vi "remoteControlArmAndGripper.vi"() -> ()   [LabVIEW 2019]
uses:
  <vilib>/ReMiSYS/ReMiSYS_myRIO-mini/SubVI/gamepadF710/F710.ctl
  <vilib>/ReMiSYS/ReMiSYS_myRIO-mini/SubVI/gamepadF710/stick.ctl
  <vilib>/ReMiSYS/ReMiSYS_myRIO-mini/SubVI/gamepadF710/gamepadF710.lvclass
  <vilib>/Platform/TimedLoop/XDataNode/timing_clust.ctl
  <vilib>/Platform/TimedLoop/XDataNode/nitl_modes.ctl
  <vilib>/Platform/TimedLoop/XDataNode/wakeup.ctl
  <vilib>/ReMiSYS/ReMiSYS_myRIO-mini/SubVI/SYS/servoPort.ctl
  <vilib>/myRIO/Common/Instrument Driver Framework/myRIO v1.0/UART/vis/myRIO v1.0 Close UART.vi
  <vilib>/myRIO/Common/Instrument Driver Framework/Utilities/vis/FPGA Ref Manager.vi
  <vilib>/myRIO/Common/Instrument Driver Framework/myRIO v1.0/myRIO v1.0 Reset FPGA.vi
  <vilib>/myRIO/Common/Instrument Driver Framework/myRIO v1.0/IRQ/vis/myRIO v1.0 IRQ Info FGV.vi
  <vilib>/myRIO/Common/Instrument Driver Framework/myRIO v1.0/IRQ/vis/myRIO v1.0 Timer IRQ Info FGV.vi
  <vilib>/myRIO/Common/Instrument Driver Framework/myRIO v1.0/IRQ/vis/myRIO v1.0 ISR Agent.vi
  <vilib>/myRIO/Instrument Drivers/Utilities/vis/Reset Index.vi
  <vilib>/myRIO/Common/Instrument Driver Framework/myRIO v1.0/Resource Manager/vis/myRIO v1.0 Block Write Resource Manager.vi
  <vilib>/Platform/TimedLoop/XDataNode/XDataNode.xnode
  <vilib>/Platform/TimedLoop/XDataNode/XDNodeRunTimeDep.lvlib
  <vilib>/myRIO/Instrument Drivers/Utilities/Utilities.lvlib
panel:
  out "F710 button info.LogiB":bool
  in  "speed 1~10":dbl=10.0
  out "shooterPitch":dbl
  out "ClipCtrl":bool[](array[boolean])
  out "Speed Array":dbl[](array[numeric])
  in  "stop Control?":bool
  out "F710":T1
  out "ENC [L, R, B] (deg)":dbl[](array[numeric])
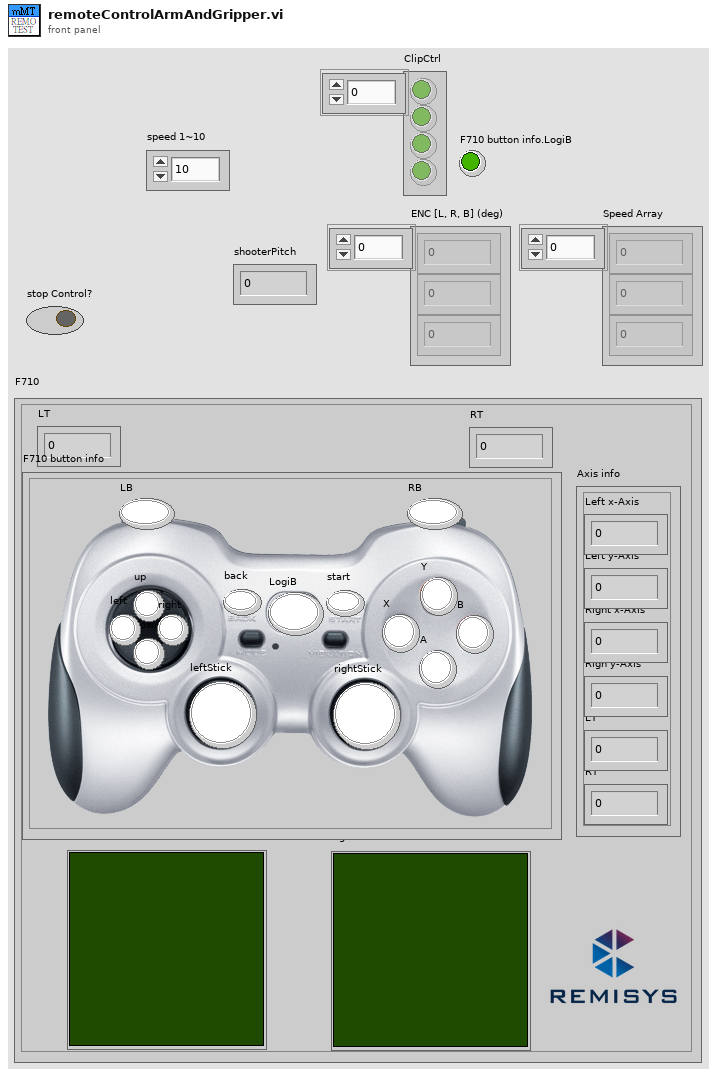
[diagram p1: front panel]
types:
  T1 = typedef "F710.ctl" = cluster{"RT":u8, "LT":u8, "RightStick":T2, "LeftStick":T2, "Axis info":cluster{"Left x-Axis":i8, "Left y-Axis":i8, "Right x-Axis":i8, "Righ y-Axis":i8, "LT":u8, "RT":u8}, "F710 button info":cluster{"RB":bool, "LB":bool, "rightStick":bool, "leftStick":bool, "start":bool, "back":bool, "right":bool, "left":bool, "down":bool, "up":bool, "Y":bool, "X":bool, "B":bool, "A":bool, "LogiB":bool}}
  T2 = typedef "stick.ctl" = cluster{"X":dbl, "Y":dbl}[]
  T3 = typedef "servoPort.ctl" = enum16{"S1", "S2", "S3", "S4", "S5", "S6", "S7", "S8", "S9"}
  T4 = typedef "XDNodeRunTimeDep.lvlib/timing_clust.ctl" = cluster{"Expected End [f-1]":u64, "Actual End [f-1]":u64, "Finished Late? [f-1]":bool, "Expected End [i-1]":u64, "Actual End [i-1]":u64, "Finished Late? [i-1]":bool, "Expected Start [i]":u64, "Actual Start [i]":u64, "Expected Start [f]":u64, "Actual Start [f]":u64, "Source Name":string, "Structure Name":string, "Period":i64, "Deadline":i64, "Offset":i64, "Start":i64, "Priority":i32, "Timeout":i32, "Mode":T5, "Wakeup Reason":T6, "Error":errorcluster, "Source Type":string, "Secondary Source Type":string, "Global End Time":u64, "Global Start Time":u64, "Frame Duration":u64, "Iteration Duration":u64, "Assigned CPU":i32, "I/O Scan Engine Mode":u32}
  T5 = typedef "XDNodeRunTimeDep.lvlib/nitl_modes.ctl" = enum32{"No Change", "Process missed periods, maintain original phase", "Discard missed periods, maintain original phase", "Process missed periods, ignore original phase", "Discard missed periods, ignore original phase"}
  T6 = typedef "XDNodeRunTimeDep.lvlib/wakeup.ctl" = enum32{"Normal", "Aborted", "Asynchronous wakeup", "Timing source error", "Timed loop error", "Timeout"}
  T7 = typedef "miniRef.ctl" = cluster{"Custom FPGA Reference":refnum<k20>, "error out":errorcluster}
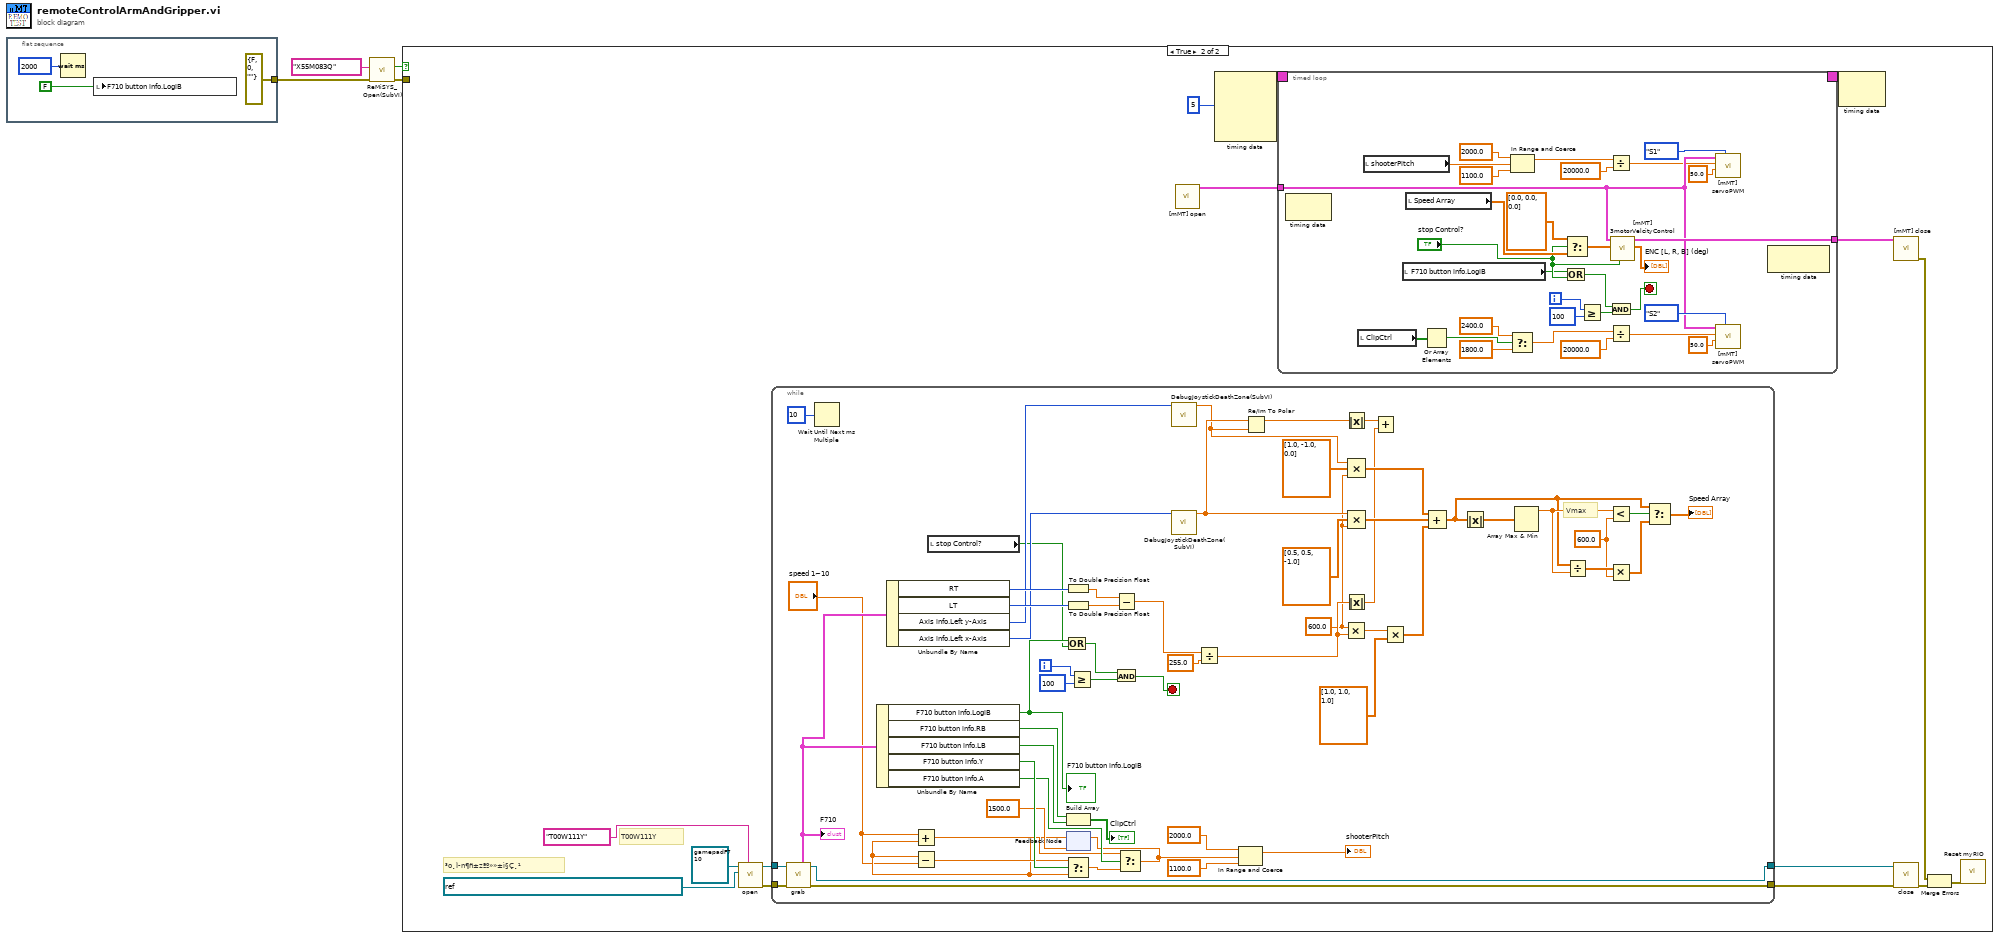
[diagram p0: block diagram]
diagram:
  n1 = flat-sequence {
    tunnel: [errorcluster {"status"=FALSE, "code"=0, "source"=""} ("error in (no error)")] -> w1
    frame #0 {
      n2 = Wait (ms)(milliseconds to wait=u32 2000) -> ()  [unwired: 1 out]
      n3 = local write "F710 button info.LogiB"(FALSE ("x .or. y?")) -> ()
    }
  }
  n4 = call <vilib>:"ReMiSYS_Open(SubVI).vi"("error in (no error)"=w1, "ReMiSYS Key"="X55M083Q") -> ("error out"=w4:errorcluster, "Correct Key?"=w3:bool)  [unwired: 8 in]
  n5 = case shown="True" w3 {
    tunnel: w4 -> [_ _]
    frame False {
    }
    frame True {
      # "T00W111Y"
      # "³o¸Ì­n¶ñ±zªº»»±ì§Ç¸¹"
      n6 = call <vilib>:"open.vi"("INPUT S/N"="T00W111Y", "VISA resource name"=refnum<visa-resource-name> "USB0::0x046D::0xC21F::A6269818::RAW", "gamepadF710 in"=refnum<class "gamepadF710.lvclass"> refnum) -> ("error out"=w13:errorcluster, "gamepadF710 out"=w17:refnum<class "gamepadF710.lvclass">)  [unwired: 7 in]
      n7 = while {
        tunnel: w17 -> [w80]
        tunnel: [w79] -> w16
        tunnel: w13 -> [w52]
        tunnel: [w51] -> w12
        i -> [w26]
        stop <- w23 stop-if-true
        w46 = 600.0 ("y")
        w42 = 600.0 ("tiltScale")
        # "Vmax"
        n8 = call <vilib>:"grab.vi"("error in (no error)"=w52, "gamepadF710 in"=w80) -> ("error out"=w51:errorcluster, "gamepadF710 out"=w79:refnum<class "gamepadF710.lvclass">, "F710"=w67:T1)  [unwired: 6 in]
        "F710" <- w67
        n9 = Wait Until Next ms Multiple(millisecond multiple=u32 10) -> ()  [unwired: 1 out]
        n10 = Unbundle By Name(w67) -> ("F710 button info.LogiB"=w29:bool, "F710 button info.RB"=w66:bool, "F710 button info.LB"=w65:bool, "F710 button info.Y"=w41:bool, "F710 button info.A"=w40:bool)
        "F710 button info.LogiB" <- w29
        n11 = Unbundle By Name(w67) -> ("RT"=w71:u8, "LT"=w69:u8, "Axis info.Left y-Axis"=w63:i8, "Axis info.Left x-Axis"=w62:i8)
        n12 = local read "stop Control?"() -> (w28:bool)
        n13 = Or(x=w29, y=w28) -> (x .or. y?=w27:bool)
        n14 = To Double Precision Float(number=w71) -> (double precision float=w70:dbl)
        n15 = To Double Precision Float(number=w69) -> (double precision float=w68:dbl)
        n16 = Build Array(w66, w65) -> (→"ClipCtrl":bool[])
        n17 = feedback #1(1500.0) -> (w35:dbl)
        n18 = Add(x="speed 1~10", y=w35) -> (x+y=w39:dbl)
        n19 = Subtract(x=w35, y="speed 1~10") -> (x-y=w37:dbl)
        n20 = Select(t=w37, s=w41, f=w35) -> (s? t:f=w38:dbl)
        n21 = Greater Or Equal?(x=w26, y=100) -> (x >= y?=w24:bool)
        n22 = Subtract(x=w70, y=w68) -> (x-y=w61:dbl)
        n23 = And(x=w27, y=w24) -> (x .and. y?=w23:bool)
        n24 = Select(t=w39, s=w40, f=w38) -> (s? t:f=w31:dbl)
        n25 = feedback-in #1(w31) -> ()
        n26 = call <vilib>:"DebugJoystickDeathZone(SubVI).vi"("Axis_Info"=w63) -> ("ValueOut 1~-1"=w58:dbl)  [unwired: 10 in]
        n27 = call <vilib>:"DebugJoystickDeathZone(SubVI).vi"("Axis_Info"=w62) -> ("ValueOut 1~-1"=w59:dbl)  [unwired: 10 in]
        n28 = Divide(x=w61, y=255.0) -> (x/y=w57:dbl)
        n29 = In Range and Coerce(upper limit=2000.0, x=w31, lower limit=1100.0) -> (coerced(x)=→"shooterPitch":dbl)  [unwired: 1 out]
        n30 = Re/Im To Polar(2:w58, 3:w59) -> (1:w56:dbl)  [unwired: 1 out]
        n31 = Multiply(x=w42, y=w57) -> (x*y=w43:dbl)
        n32 = Absolute Value(x=w56) -> (abs(x)=w55:dbl)
        n33 = Absolute Value(x=w57) -> (abs(x)=w54:dbl)
        n34 = Compound Arithmetic op=MULTIPLY(w58, dbl[] [1.0, -1.0, 0.0], w42) -> (w74:dbl[])
        n35 = Compound Arithmetic op=MULTIPLY(w59, dbl[] [0.5, 0.5, -1.0], w42) -> (w73:dbl[])
        n36 = Add(x=w55, y=w54) -> ()  [unwired: 1 out]
        n37 = Multiply(x=w43, y=dbl[] [1.0, 1.0, 1.0]) -> (x*y=w72:dbl[])
        n38 = Compound Arithmetic op=ADD(w74, w73, w72) -> (w48:dbl[])
        n39 = Absolute Value(x=w48) -> (abs(x)=w53:dbl[])
        n40 = Array Max & Min(array=w53) -> (max value=w49:dbl)  [unwired: 3 out]
        n41 = Divide(x=w48, y=w49) -> (x/y=w47:dbl[])
        n42 = Less?(x=w49, y=w46) -> (x < y?=w50:bool)
        n43 = Multiply(x=w47, y=w46) -> (x*y=w45:dbl[])
        n44 = Select(t=w48, s=w50, f=w45) -> (s? t:f=→"Speed Array":dbl[])
      }
      n45 = call <vilib>:"[mMT] open.vi"() -> ("miniOut"=w20:T7)  [unwired: 9 in, 2 out]
      n46 = node-c288(i64 5 ("Period")) -> (w22:T4)  [unwired: 3 in]
      n47 = timed-loop {
        tunnel: w20 -> [w101]
        timing: w22 -> [_]
        timing-out: [_] -> w21
        tunnel: [w110] -> w19
        i -> [w83]
        stop <- w81 stop-if-true
        n48 = node-c288() -> ()  [unwired: 1 in, 1 out]
        n49 = local read "ClipCtrl"() -> (w98:bool[])
        n50 = local read "shooterPitch"() -> (w88:dbl)
        n51 = local read "F710 button info.LogiB"() -> (w82:bool)
        n52 = local read "Speed Array"() -> (w108:dbl[])
        n53 = Or Array Elements(Boolean array=w98) -> (logical OR=w97:bool)
        n54 = Select(t=2400.0 ("y"), s=w97, f=1800.0 ("y")) -> (s? t:f=w90:dbl)
        n55 = In Range and Coerce(upper limit=2000.0, x=w88, lower limit=1100.0) -> (coerced(x)=w93:dbl)  [unwired: 1 out]
        n56 = Or(x=w82, y="stop Control?") -> (x .or. y?=w84:bool)
        n57 = Select(t=dbl[] [0.0, 0.0, 0.0], s="stop Control?", f=w108) -> (s? t:f=w106:dbl[])
        n58 = Greater Or Equal?(x=w83, y=100) -> (x >= y?=w85:bool)
        n59 = Divide(x=w93, y=20000.0) -> (x/y=w94:dbl)
        n60 = Divide(x=w90, y=20000.0) -> (x/y=w89:dbl)
        n61 = And(x=w84, y=w85) -> (x .and. y?=w81:bool)
        n62 = call <vilib>:"[mMT] 3motorVelcityControl.vi"("reset?"="stop Control?", "Speed [L, R, B] (deg/s)"=w106, "miniOut in"=w101) -> ("ENC [L, R, B] (deg)"=→"ENC [L, R, B] (deg)":dbl[], "miniOut out"=w110:T7)  [unwired: 5 in, 2 out]
        n63 = call <vilib>:"[mMT] servoPWM.vi"("servoPort"=servoPort."S1", "Frequency"=50.0, "DutyCycle"=w94, "miniOut in"=w101) -> ()  [unwired: 6 in, 2 out]
        n64 = call <vilib>:"[mMT] servoPWM.vi"("servoPort"=servoPort."S2", "Frequency"=50.0, "DutyCycle"=w89, "miniOut in"=w101) -> ()  [unwired: 6 in, 2 out]
        n65 = node-c288() -> ()  [unwired: 1 in, 1 out]
      }
      n66 = node-c288(w21) -> ()  [unwired: 1 out]
      n67 = call <vilib>:"[mMT] close.vi"("miniOut in"=w19) -> ("error out"=w11:errorcluster)  [unwired: 10 in]
      n68 = call <vilib>:"close.vi"("error in (no error)"=w12, "gamepadF710 in"=w16) -> ("error out"=w10:errorcluster)  [unwired: 8 in, 1 out]
      n69 = Merge Errors(w11, w10) -> (w9:errorcluster)
      n70 = call <vilib>:"Reset myRIO.vi"("error in (no error)"=w9) -> ()  [unwired: 10 in, 1 out]
    }
  }
